vi "Try Match Response.vi"(8 "error in":errorcluster, 10 "ICAN CC Frame":refnum<class "ICAN CC Frame.lvclass">, 11 "Block Upload Initiate in":refnum<class "Block Upload Initiate Transfer.lvclass">) -> (0 "error out":errorcluster, 2 "Match":bool, 3 "SDO Transfer out":refnum<class "SDO Transfer.lvclass">)   [LabVIEW 2020, in "CANopen.lvlib" / "SDO Manager.lvlib" / "Block Upload Initiate Transfer.lvclass"]
uses:
  Block Upload Initiate Transfer.lvclass
  SDO Transfer/SDO Transfer.lvclass
  HAL/Source/Interfaces/ICAN CC Frame/ICAN CC Frame.lvclass
  Block Upload Initiate Transfer.lvclass/Block Upload Initiate Transfer.ctl
  HAL/Source/Interfaces/ICommunicate/ICommunicate.lvclass
  D:/git/CANopen-LabVIEW/source/SDO/SDO Manager/SDO Transfer/SDO Transfer.lvclass
  D:/git/CANopen-LabVIEW/source/SDO/SDO Manager/Block Upload Initiate Transfer/Block Upload Initiate Transfer.lvclass
  CANopen Message/CANopen Message.lvclass
  Upload Transfer/Upload Transfer.lvclass
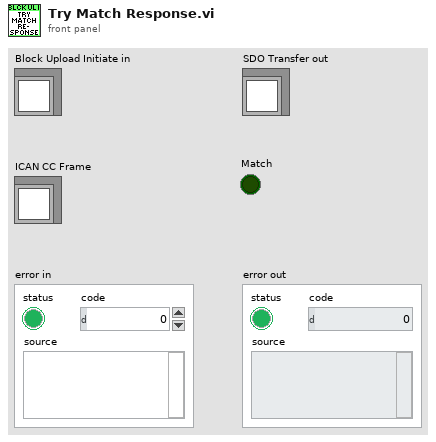
[diagram p1: front panel]
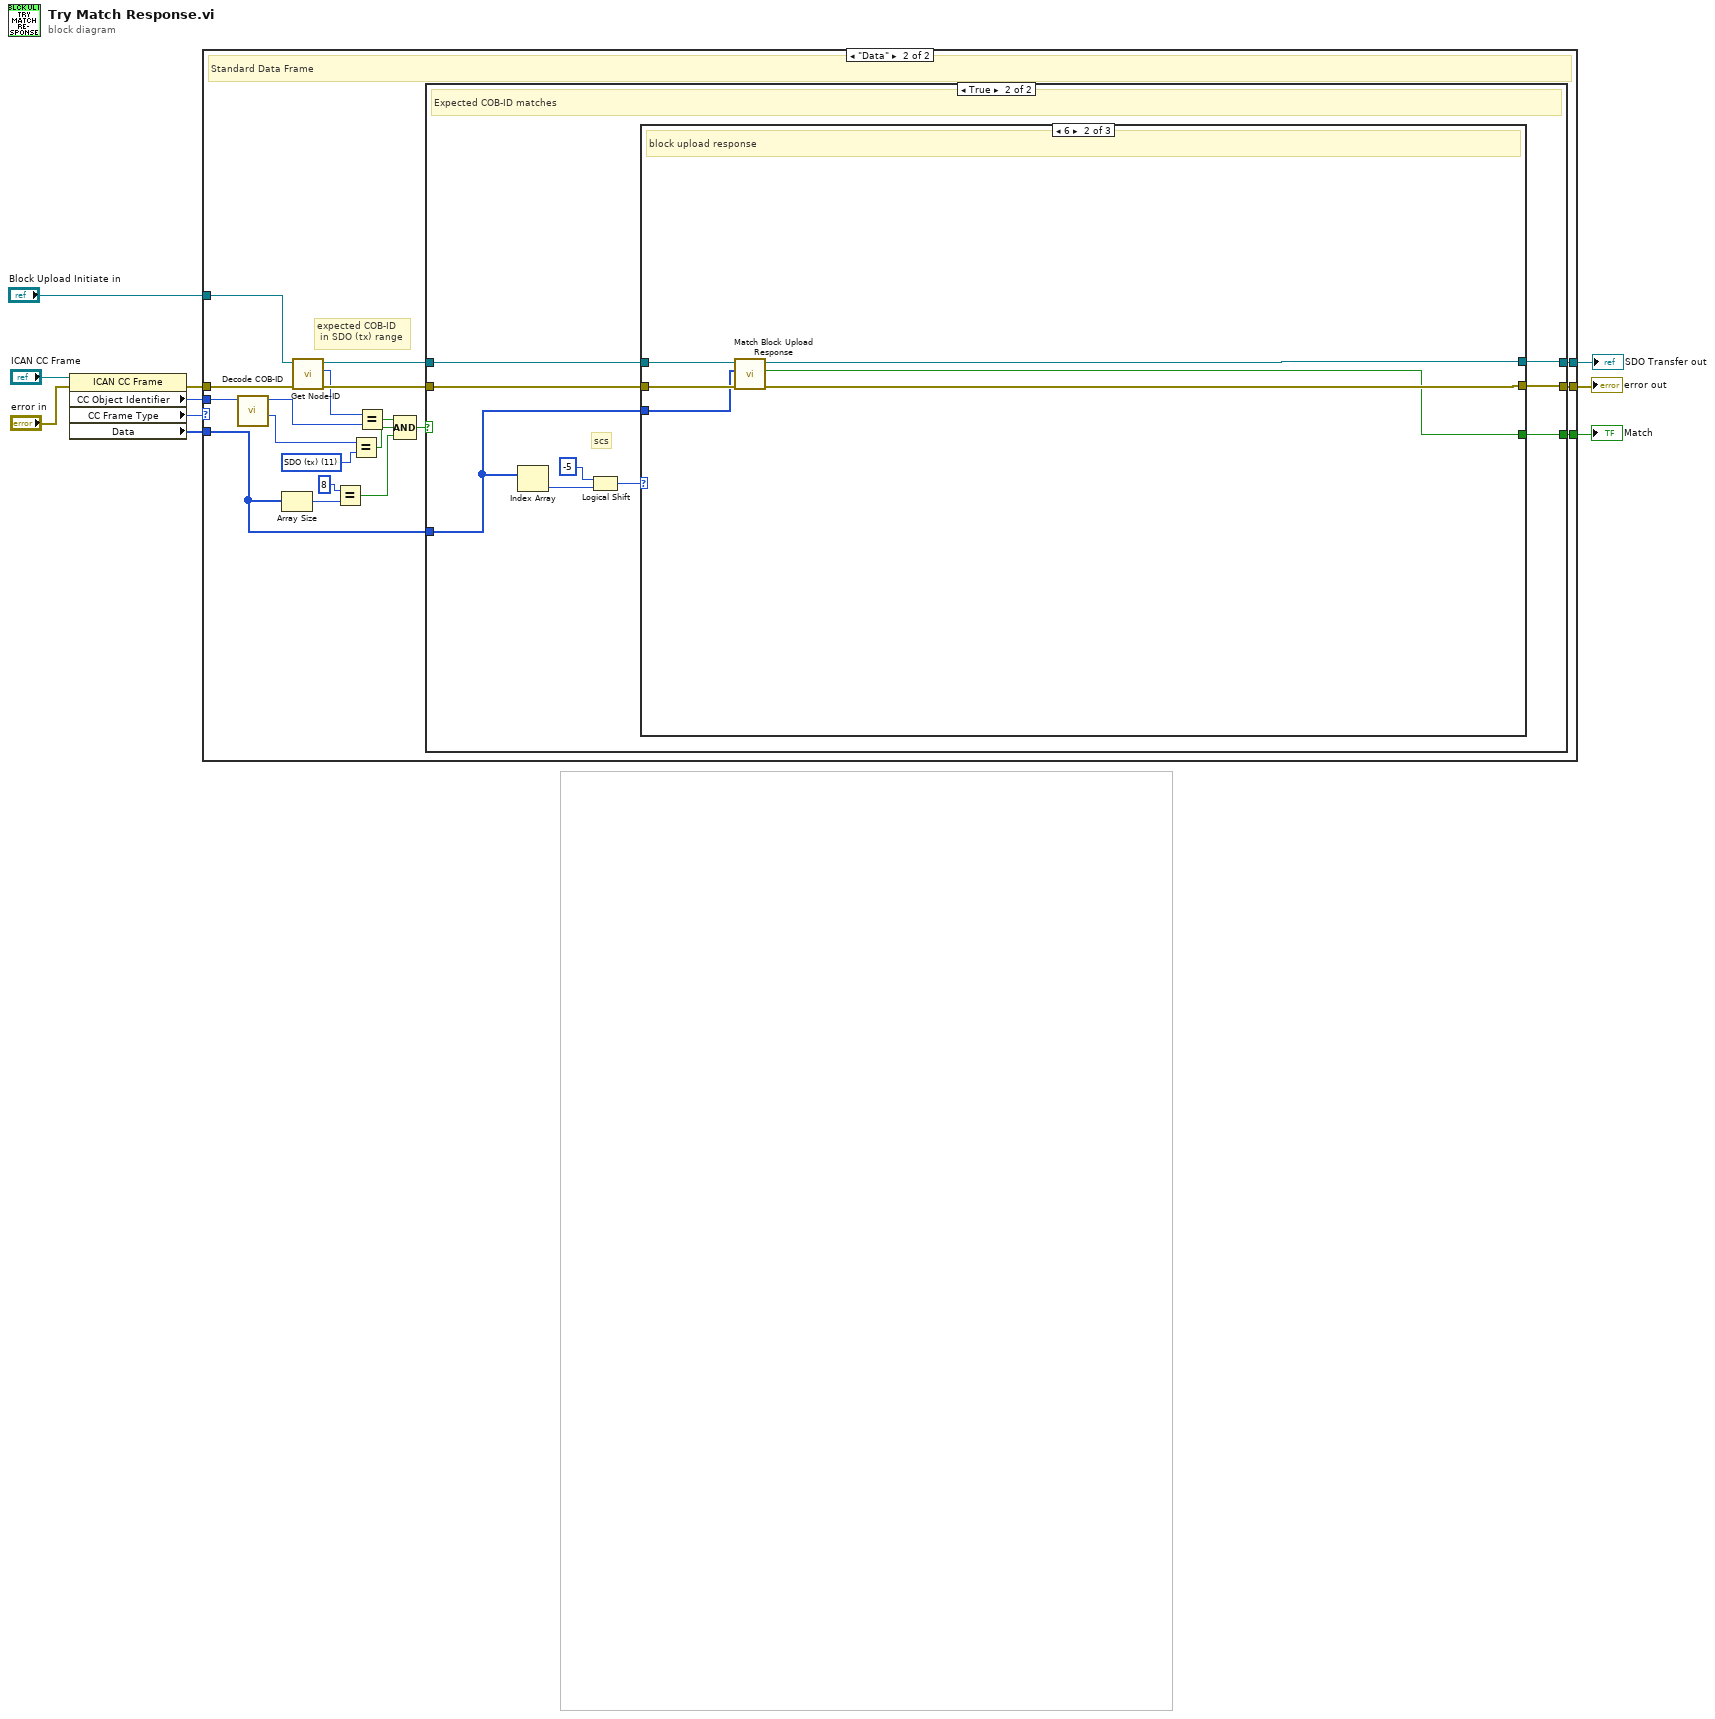
[diagram p0: block diagram]
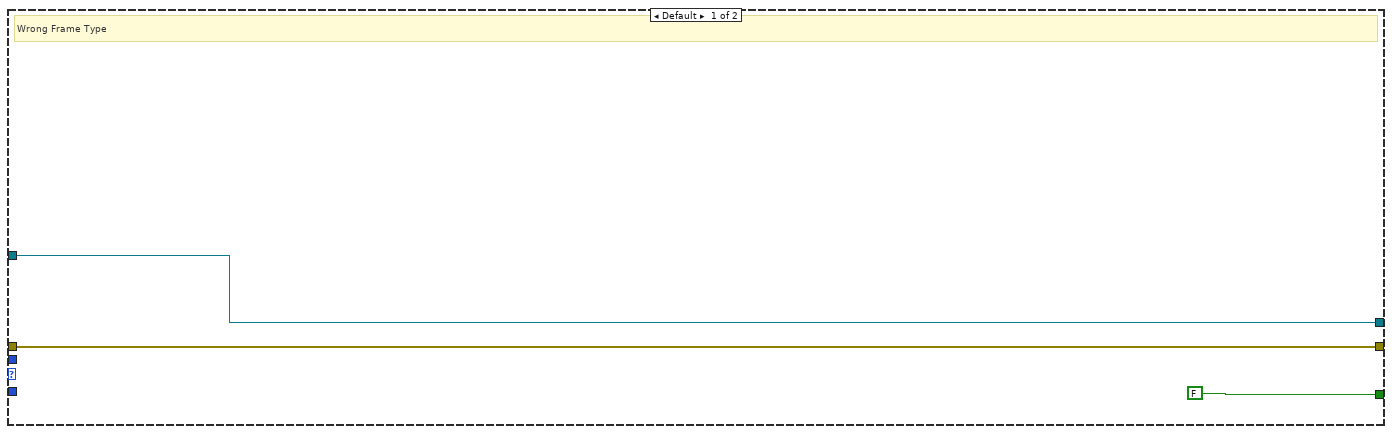
[diagram p2: hidden frame]
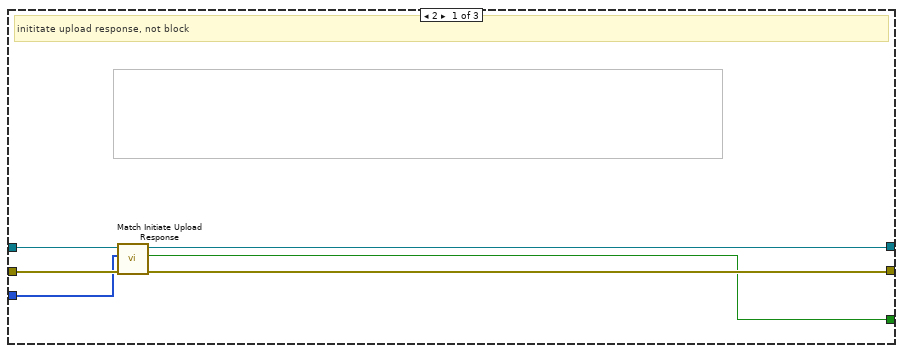
[diagram p4: hidden frame]
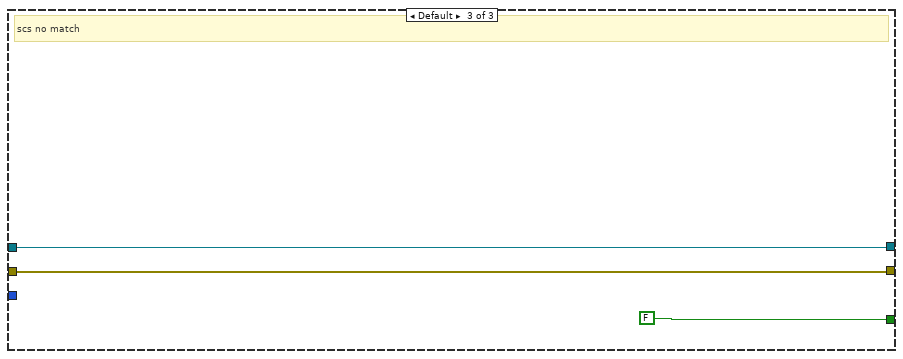
[diagram p5: hidden frame]
diagram:
  n1 = property class="ICAN CC Frame"(reference="ICAN CC Frame", error in="error in") -> (error out=w10:errorcluster, "CC Object Identifier"=w9:u32, "CC Frame Type"=w7:enum8{"Data", "Remote", "Error", "Overload"}, "Data"=w8:u8[])  [unwired: 1 out]
  n2 = case shown="\"Data\"" w7 {
    tunnel: w10 -> [w12 w32]
    tunnel: "Block Upload Initiate in" -> [w11 w31]
    tunnel: [w11 w28] -> w2
    tunnel: [w12 w27] -> w3
    tunnel: [FALSE w26] -> w1
    tunnel: w9 -> [_ w25]
    tunnel: w8 -> [_ w14]
    frame Default {
      # "Wrong Frame Type"
    }
    frame "Data" {
      w22 = u8 11 items=["NMT"=0, "EMCY/SYNC"=1, "TIME"=2, "PDO1 (tx)"=3, "PDO1 (rx)"=4, "PDO2 (tx)"=5, "PDO2 (rx)"=6, "PDO3 (tx)"=7, "PDO3 (rx)"=8, "PDO4 (tx)"=9, "PDO4 (rx)"=10, "SDO (tx)"=11, "SDO (rx)"=12, "NMT error control"=14] ("Function Code")
      # "expected COB-ID\n in SDO (tx) range"
      # "Standard Data Frame"
      n3 = call "Decode COB-ID.vi"("COD-ID"=w25) -> ("Function Code"=w21:u8, "Node-ID"=w24:u8)  [unwired: 9 in]
      n4 = Array Size(array=w14) -> (size(s)=w20:i32)
      n5 = call "Get Node-ID.vi"("error in"=w32, "SDO Transfer in"=w31) -> ("error out"=w29:errorcluster, "Node-ID"=w23:u8, "SDO Transfer out"=w30:refnum<class "Block Upload Initiate Transfer.lvclass">)  [unwired: 7 in]
      n6 = Equal?(x=8, y=w20) -> (x = y?=w15:bool)
      n7 = Equal?(x=w21, y=w22) -> (x = y?=w16:bool)
      n8 = Equal?(x=w23, y=w24) -> (x = y?=w17:bool)
      n9 = Compound Arithmetic op=AND(w17, w16, w15) -> (w18:bool)
      n10 = case shown="True" w18 {
        tunnel: w30 -> [w34 w42]
        tunnel: w29 -> [w33 w41]
        tunnel: [w34 w38] -> w28
        tunnel: [w33 w39] -> w27
        tunnel: w14 -> [_ w35]
        tunnel: [_ w37] -> w26
        frame False {
        }
        frame True {
          # "scs"
          # "Expected COB-ID matches"
          n11 = Index Array(array=w35) -> (element=w36:u8)  [unwired: 1 in]
          n12 = Logical Shift(y=i16 -5, x=w36) -> (x << y=w40:u8)
          n13 = case shown="6" w40 {
            tunnel: w42 -> [w49 w51 w57]
            tunnel: w41 -> [w48 w55 w58]
            tunnel: [w45 w54 w57] -> w38
            tunnel: [w46 w53 w58] -> w39
            tunnel: [w44 w52 FALSE] -> w37
            tunnel: w35 -> [w47 w50 _]
            frame 2 {
              # "inititate upload response, not block"
              n14 = call "Match Initiate Upload Response.vi"("error in"=w48, "Frame Data"=w47, "SDO Transfer in"=w49) -> ("error out"=w46:errorcluster, "Match"=w44:bool, "SDO Transfer out"=w45:refnum<class "SDO Transfer.lvclass">)  [unwired: 6 in]
            }
            frame 6 {
              # "block upload response"
              n15 = call "Match Block Upload Response.vi"("error in"=w55, "Frame Data"=w50, "Block Upload Initiate in"=w51) -> ("error out"=w53:errorcluster, "Match"=w52:bool, "SDO Transfer out"=w54:refnum<class "SDO Transfer.lvclass">)  [unwired: 6 in]
            }
            frame Default {
              # "scs no match"
            }
          }
        }
      }
    }
  }
  "SDO Transfer out" <- w2
  "error out" <- w3
  "Match" <- w1
